vi "Compute normals for 3D visualization vertices.vi"(11 "Vertex data":T1) -> (3 "Vertex data new normals":T1)   [LabVIEW 2015, in "Morph Cortical Surfaces.lvlib"]
doc: "Compute right-handed normals from triangles using cross-product."
uses:
  Morph Cortical Surfaces.lvlib
  Vertex data control.ctl
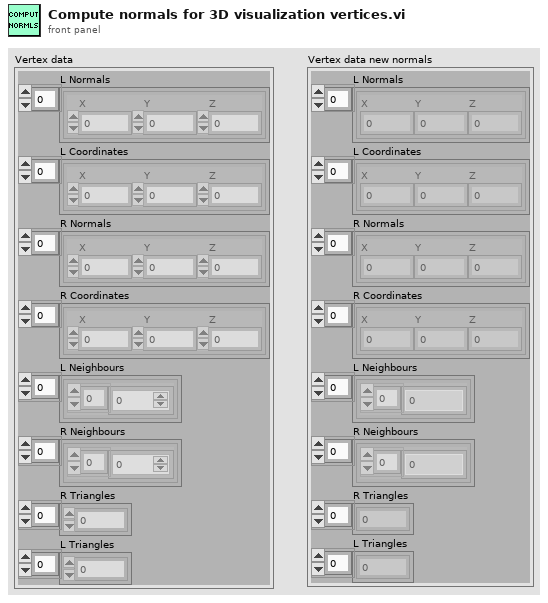
[diagram p1: front panel]
types:
  T1 = typedef "Morph Cortical Surfaces.lvlib/Vertex data control.ctl" = cluster{"L Normals":cluster{"X":sgl, "Y":sgl, "Z":sgl}[], "L Coordinates":cluster{"X":sgl, "Y":sgl, "Z":sgl}[], "R Normals":cluster{"X":sgl, "Y":sgl, "Z":sgl}[], "R Coordinates":cluster{"X":sgl, "Y":sgl, "Z":sgl}[], "L Neighbours":cluster{i32[]}[], "R Neighbours":cluster{i32[]}[], "R Triangles":i32[], "L Triangles":i32[]}
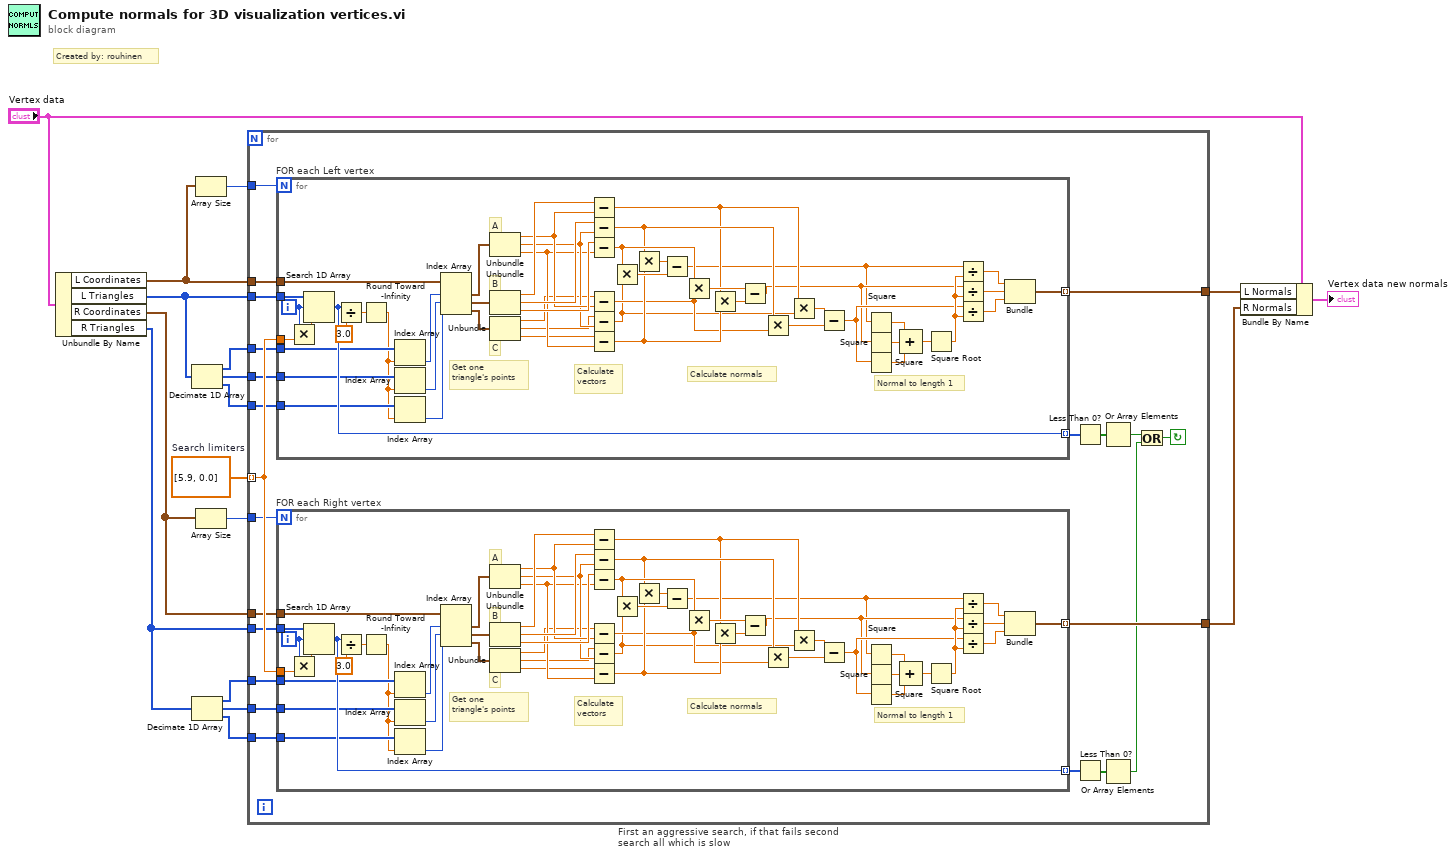
[diagram p0: block diagram]
diagram:
  w17 = dbl[] [5.9, 0.0]  # Search limiters
  # "Created by: rouhinen"
  n1 = Unbundle By Name("Vertex data") -> ("L Coordinates"=w8:cluster{"X":sgl, "Y":sgl, "Z":sgl}[], "L Triangles"=w4:i32[], "R Coordinates"=w14:cluster{"X":sgl, "Y":sgl, "Z":sgl}[], "R Triangles"=w15:i32[])
  n2 = Decimate 1D Array(w4) -> (w7:i32[], w5:i32[], w6:i32[])
  n3 = Decimate 1D Array(w15) -> (w11:i32[], w13:i32[], w12:i32[])
  n4 = Array Size(array=w8) -> (size(s)=w9:i32)
  n5 = Array Size(array=w14) -> (size(s)=w10:i32)
  n6 = for "First an aggressive search, if that fails second search all which is slow" {
    tunnel: [w38] -> w3
    tunnel: w4 -> [w37]
    tunnel: w5 -> [w36]
    tunnel: w6 -> [w35]
    tunnel: w7 -> [w34]
    tunnel: w8 -> [w33]
    tunnel: w9 -> [w32]
    tunnel: w10 -> [w31]
    tunnel: w11 -> [w30]
    tunnel: w12 -> [w29]
    tunnel: w13 -> [w28]
    tunnel: w14 -> [w27]
    tunnel: w15 -> [w26]
    tunnel: [w25] -> w16
    tunnel: w17 -> [w39] mode=indexing
    stop <- w18 continue-if-true
    n7 = for "FOR each Left vertex" {
      N: w32 -> [_]
      tunnel: w33 -> [w136]
      tunnel: [w135] -> w38 mode=indexing
      tunnel: w37 -> [w132]
      tunnel: w36 -> [w127]
      tunnel: w35 -> [w126]
      tunnel: w34 -> [w112]
      tunnel: w39 -> [w107]
      tunnel: [w141] -> w24 mode=indexing
      i -> [w108]
      # "Get one\ntriangle's points"
      # "Calculate normals"
      # "Calculate\nvectors"
      # "Normal to length 1"
      # "B"
      # "C"
      # "A"
      n8 = Multiply(x=w108, y=w107) -> (x*y=w106:dbl)
      n9 = Search 1D Array(1D array=w132, element=w108, start index (0)=w106) -> (index of element=w141:i32)
      n10 = Divide(x=w141, y=3.0) -> (x/y=w130:dbl)
      n11 = Round Toward -Infinity(1:w130) -> (0:w109:dbl)
      n12 = Index Array(array=w112, index=w109) -> (element=w111:i32)
      n13 = Index Array(array=w127, index=w109) -> (element=w129:i32)
      n14 = Index Array(array=w126, index=w109) -> (element=w128:i32)
      n15 = Index Array(array=w136, index #1=w111, index #2=w129, index #3=w128) -> (element #1=w110:cluster{"X":sgl, "Y":sgl, "Z":sgl}, element #2=w113:cluster{"X":sgl, "Y":sgl, "Z":sgl}, element #3=w133:cluster{"X":sgl, "Y":sgl, "Z":sgl})
      n16 = Unbundle(w110) -> ("X"=w122:sgl, "Y"=w121:sgl, "Z"=w120:sgl)
      n17 = Unbundle(w113) -> ("X"=w125:sgl, "Y"=w124:sgl, "Z"=w123:sgl)
      n18 = Unbundle(w133) -> ("X"=w119:sgl, "Y"=w118:sgl, "Z"=w117:sgl)
      n19 = Subtract(x=w125, y=w122) -> (x-y=w95:sgl)
      n20 = Subtract(x=w124, y=w121) -> (x-y=w97:sgl)
      n21 = Subtract(x=w123, y=w120) -> (x-y=w102:sgl)
      n22 = Subtract(x=w119, y=w122) -> (x-y=w96:sgl)
      n23 = Subtract(x=w118, y=w121) -> (x-y=w94:sgl)
      n24 = Subtract(x=w117, y=w120) -> (x-y=w103:sgl)
      n25 = Multiply(x=w102, y=w94) -> (x*y=w104:sgl)
      n26 = Multiply(x=w97, y=w103) -> (x*y=w105:sgl)
      n27 = Subtract(x=w105, y=w104) -> (x-y=w91:sgl)
      n28 = Multiply(x=w102, y=w96) -> (x*y=w101:sgl)
      n29 = Multiply(x=w95, y=w103) -> (x*y=w100:sgl)
      n30 = Subtract(x=w101, y=w100) -> (x-y=w92:sgl)
      n31 = Multiply(x=w97, y=w96) -> (x*y=w98:sgl)
      n32 = Multiply(x=w95, y=w94) -> (x*y=w99:sgl)
      n33 = Subtract(x=w99, y=w98) -> (x-y=w93:sgl)
      n34 = Square(x=w91) -> (x^2=w138:sgl)
      n35 = Square(x=w92) -> (x^2=w137:sgl)
      n36 = Square(x=w93) -> (x^2=w139:sgl)
      n37 = Compound Arithmetic op=ADD(w138, w137, w139) -> (w140:sgl)
      n38 = Square Root(x=w140) -> (sqrt(x)=w134:sgl)
      n39 = Divide(x=w91, y=w134) -> (x/y=w116:sgl)
      n40 = Divide(x=w92, y=w134) -> (x/y=w115:sgl)
      n41 = Divide(x=w93, y=w134) -> (x/y=w114:sgl)
      n42 = Bundle(w116, w115, w114) -> (w135:cluster{sgl, sgl, sgl})  [unwired: 1 in]
    }
    n43 = for "FOR each Right vertex" {
      N: w31 -> [_]
      tunnel: w27 -> [w85]
      tunnel: [w84] -> w25 mode=indexing
      tunnel: w26 -> [w81]
      tunnel: w28 -> [w76]
      tunnel: w29 -> [w75]
      tunnel: w30 -> [w61]
      tunnel: w39 -> [w56]
      tunnel: [w90] -> w23 mode=indexing
      i -> [w57]
      # "Get one\ntriangle's points"
      # "Calculate normals"
      # "Calculate\nvectors"
      # "Normal to length 1"
      # "B"
      # "C"
      # "A"
      n44 = Multiply(x=w57, y=w56) -> (x*y=w55:dbl)
      n45 = Search 1D Array(1D array=w81, element=w57, start index (0)=w55) -> (index of element=w90:i32)
      n46 = Divide(x=w90, y=3.0) -> (x/y=w79:dbl)
      n47 = Round Toward -Infinity(1:w79) -> (0:w58:dbl)
      n48 = Index Array(array=w61, index=w58) -> (element=w60:i32)
      n49 = Index Array(array=w76, index=w58) -> (element=w78:i32)
      n50 = Index Array(array=w75, index=w58) -> (element=w77:i32)
      n51 = Index Array(array=w85, index #1=w60, index #2=w78, index #3=w77) -> (element #1=w59:cluster{"X":sgl, "Y":sgl, "Z":sgl}, element #2=w62:cluster{"X":sgl, "Y":sgl, "Z":sgl}, element #3=w82:cluster{"X":sgl, "Y":sgl, "Z":sgl})
      n52 = Unbundle(w59) -> ("X"=w71:sgl, "Y"=w70:sgl, "Z"=w69:sgl)
      n53 = Unbundle(w62) -> ("X"=w74:sgl, "Y"=w73:sgl, "Z"=w72:sgl)
      n54 = Unbundle(w82) -> ("X"=w68:sgl, "Y"=w67:sgl, "Z"=w66:sgl)
      n55 = Subtract(x=w74, y=w71) -> (x-y=w44:sgl)
      n56 = Subtract(x=w73, y=w70) -> (x-y=w46:sgl)
      n57 = Subtract(x=w72, y=w69) -> (x-y=w51:sgl)
      n58 = Subtract(x=w68, y=w71) -> (x-y=w45:sgl)
      n59 = Subtract(x=w67, y=w70) -> (x-y=w43:sgl)
      n60 = Subtract(x=w66, y=w69) -> (x-y=w52:sgl)
      n61 = Multiply(x=w51, y=w43) -> (x*y=w53:sgl)
      n62 = Multiply(x=w46, y=w52) -> (x*y=w54:sgl)
      n63 = Subtract(x=w54, y=w53) -> (x-y=w40:sgl)
      n64 = Multiply(x=w51, y=w45) -> (x*y=w50:sgl)
      n65 = Multiply(x=w44, y=w52) -> (x*y=w49:sgl)
      n66 = Subtract(x=w50, y=w49) -> (x-y=w41:sgl)
      n67 = Multiply(x=w46, y=w45) -> (x*y=w47:sgl)
      n68 = Multiply(x=w44, y=w43) -> (x*y=w48:sgl)
      n69 = Subtract(x=w48, y=w47) -> (x-y=w42:sgl)
      n70 = Square(x=w40) -> (x^2=w87:sgl)
      n71 = Square(x=w41) -> (x^2=w86:sgl)
      n72 = Square(x=w42) -> (x^2=w88:sgl)
      n73 = Compound Arithmetic op=ADD(w87, w86, w88) -> (w89:sgl)
      n74 = Square Root(x=w89) -> (sqrt(x)=w83:sgl)
      n75 = Divide(x=w40, y=w83) -> (x/y=w65:sgl)
      n76 = Divide(x=w41, y=w83) -> (x/y=w64:sgl)
      n77 = Divide(x=w42, y=w83) -> (x/y=w63:sgl)
      n78 = Bundle(w65, w64, w63) -> (w84:cluster{sgl, sgl, sgl})  [unwired: 1 in]
    }
    n79 = Less Than 0?(x=w24) -> (x < 0?=w21:bool[])
    n80 = Less Than 0?(x=w23) -> (x < 0?=w22:bool[])
    n81 = Or Array Elements(Boolean array=w21) -> (logical OR=w20:bool)
    n82 = Or Array Elements(Boolean array=w22) -> (logical OR=w19:bool)
    n83 = Or(x=w20, y=w19) -> (x .or. y?=w18:bool)
  }
  n84 = Bundle By Name(cluster="Vertex data", "L Normals"=w3, "R Normals"=w16) -> (→"Vertex data new normals":T1)
